vi "Channel Config Dialog.vi"(8 "error in (no error)":errorcluster caption="错误输入（无错误）", 11 "Type":enum16{"Device", "Ch0", "Ch1"}(ring)) -> (0 "error out":errorcluster caption="错误输出", 1 "Filter":T1 {"Config"."End" format="%x"; "Config"."Start" format="%x"}, 2 "Param":T2={"Terminal"=0, "Param"={"abitbaud"=500000, "dbitbaud"=500000, "CustomBaud"=FALSE, "CustomBd"="", "Mode"=0, "Standard"=0}} {"Param"."Standard" items=["CANFD ISO", "CANFD BOSCH"]; "Param"."dbitbaud" items=["5Mbps"=5000000, "4Mbps"=4000000, "2Mbps"=2000000, "1Mbps"=1000000, "800kbps"=800000, "500kbps"=500000, "250kbps"=250000, "125kbps"=125000, "100kbps"=100000]; "Param"."abitbaud" items=["1Mbps"=1000000, "800kbps"=800000, "500kbps"=500000, "250kbps"=250000, "125kbps"=125000, "100kbps"=100000, "50kbps"=50000]; "Param"."Mode" items=["正常", "只听"]; "Terminal" items=["禁用", "启用"]}, 3 "Cancel":bool)   [LabVIEW 2011, in "CAN FD.lvlib"]
uses:
  CAN FD.lvlib
panel:
  in  "FilterSetting":bool
  in  "Filter":bool caption="启用滤波"
  in  "Input":T2={"Terminal"=0, "Param"={"abitbaud"=500000, "dbitbaud"=500000, "CustomBaud"=FALSE, "CustomBd"="", "Mode"=0, "Standard"=0}} {"Param"."Standard" items=["CANFD ISO", "CANFD BOSCH"]; "Param"."dbitbaud" items=["5Mbps"=5000000, "4Mbps"=4000000, "2Mbps"=2000000, "1Mbps"=1000000, "800kbps"=800000, "500kbps"=500000, "250kbps"=250000, "125kbps"=125000, "100kbps"=100000]; "Param"."abitbaud" items=["1Mbps"=1000000, "800kbps"=800000, "500kbps"=500000, "250kbps"=250000, "125kbps"=125000, "100kbps"=100000, "50kbps"=50000]; "Param"."Mode" items=["正常", "只听"]; "Terminal" items=["禁用", "启用"]}
  in  "Cancel":bool
  in  "OK":bool
  # "启动参数"
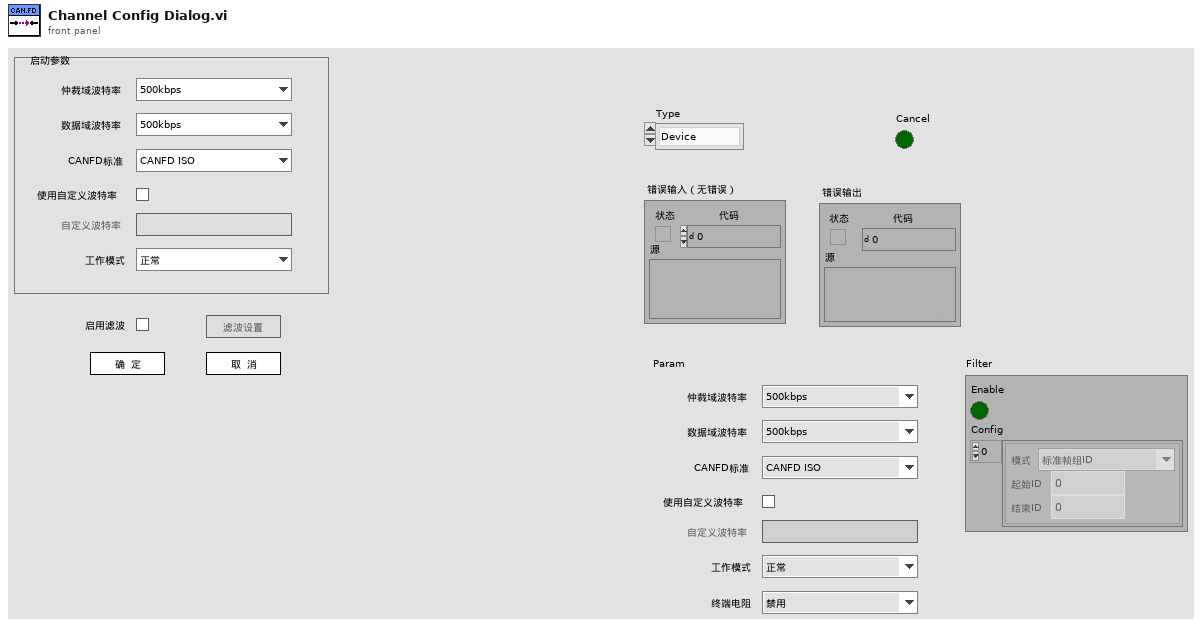
[diagram p1: front panel]
types:
  T1 = cluster{"Enable":bool, "Config":cluster{"Mode":enum16{"标准帧组ID", "标准帧明确ID", "扩展帧组ID", "扩展帧明确ID"}, "Start":u32, "End":u32}[]}
  T2 = cluster{"Terminal":u32, "Param":cluster{"abitbaud":u32, "dbitbaud":u32, "CustomBaud":bool, "CustomBd":string, "Mode":u8, "Standard":u32}}
  T3 = cluster{"Mode":enum16{"标准帧组ID", "标准帧明确ID", "扩展帧组ID", "扩展帧明确ID"}, "Start":u32, "End":u32}[]
  T4 = cluster{"Filter":bool, "Filter in":cluster{"Mode":enum16{"标准帧组ID", "标准帧明确ID", "扩展帧组ID", "扩展帧明确ID"}, "Start":u32, "End":u32}[]}
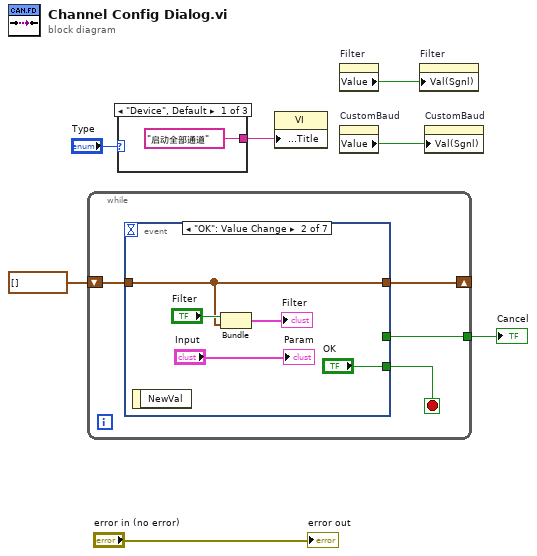
[diagram p0: block diagram]
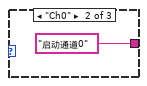
[diagram p2: hidden frame]
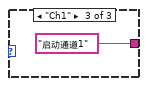
[diagram p3: hidden frame]
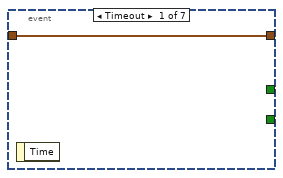
[diagram p4: hidden frame]
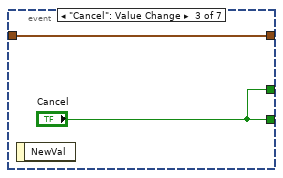
[diagram p5: hidden frame]
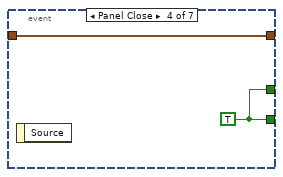
[diagram p6: hidden frame]
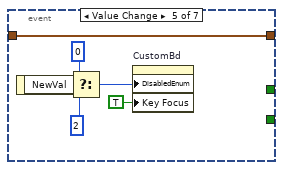
[diagram p7: hidden frame]
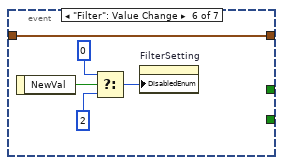
[diagram p8: hidden frame]
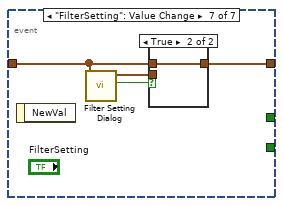
[diagram p9: hidden frame]
diagram:
  n1 = while {
    tunnel: [w10] -> w3
    shift-right: [w8] -> _
    shift-left: T3 [] ("Filter in") -> [w9]
    stop <- w11 stop-if-true
    n2 = event shown="[1] \"OK\": Value Change" {
      selector: _ -> [_ _ _ _ _ _ _]
      dyn-events: _ -> [_ _ _ _ _ _ _]
      timeout: _ -> [_ _ _ _ _ _ _]
      tunnel: [_ "OK" "Cancel" w21 _ _ _] -> w11
      tunnel: [_ _ "Cancel" w21 _ _ _] -> w10
      tunnel: w9 -> [w12 w14 w18 w20 w22 w28 w33]
      tunnel: [w12 w14 w18 w20 w22 w28 w35] -> w8
      event Timeout {
        n3 = event-data() -> ()  [unwired: 1 in, 1 out]
      }
      event "OK": Value Change {
        n4 = event-data() -> ()  [unwired: 1 in, 1 out]
        n5 = Bundle("Filter"="Filter", "Filter in"=w14) -> (→"Filter":T4)  [unwired: 1 in]
        "Param" <- "Input"
      }
      event "Cancel": Value Change {
        n6 = event-data() -> ()  [unwired: 1 in, 1 out]
      }
      event Panel Close {
        w21 = TRUE ("Cancel")
        n7 = event-data() -> ()  [unwired: 1 in, 1 out]
      }
      event "Input.Param.CustomBaud": Value Change {
        n8 = event-data() -> ("NewVal"=w23:bool)  [unwired: 1 in]
        n9 = Select(t=0, s=w23, f=2) -> (s? t:f=w25:i32)
        n10 = property on="CustomBd" class="Str"("DisabledEnum"=w25, "Key Focus"=TRUE ("键选中")) -> ()  [unwired: 2 in, 2 out]
      }
      event "Filter": Value Change {
        n11 = event-data() -> ("NewVal"=w32:bool)  [unwired: 1 in]
        n12 = Select(t=0, s=w32, f=2) -> (s? t:f=w29:i32)
        n13 = property on="FilterSetting" class="Bool"("DisabledEnum"=w29) -> ()  [unwired: 2 in, 2 out]
      }
      event "FilterSetting": Value Change {
        n14 = event-data() -> ()  [unwired: 1 in, 1 out]
        n15 = call "Filter Setting Dialog.vi"("Filter in"=w33) -> ("Cancel?"=w36:bool, "Filter out"=w34:T3)  [unwired: 9 in]
        n16 = case shown="True" w36 {
          tunnel: [w37 w38] -> w35
          tunnel: w33 -> [_ w38]
          tunnel: w34 -> [w37 _]
          frame False {
          }
          frame True {
          }
        }
      }
    }
  }
  "Cancel" <- w3
  n17 = case shown="\"Device\", Default" "Type" {
    tunnel: ["启动全部通道" "启动通道0" "启动通道1"] -> w5
    frame "Device", Default {
    }
    frame "Ch0" {
    }
    frame "Ch1" {
    }
  }
  n18 = property class="VI"("Front Panel.Title"=w5) -> ()  [unwired: 2 in, 2 out]
  n19 = property on="Filter" class="Bool (严格)"() -> ("Value"=w2:bool)  [unwired: 2 in, 2 out]
  n20 = property on="CustomBaud" class="Bool (严格)"() -> ("Value"=w4:bool)  [unwired: 2 in, 2 out]
  n21 = property on="Filter" class="Bool (严格)"("Val(Sgnl)"=w2) -> ()  [unwired: 2 in, 2 out]
  n22 = property on="CustomBaud" class="Bool (严格)"("Val(Sgnl)"=w4) -> ()  [unwired: 2 in, 2 out]
  "error out" <- "error in (no error)"
